vi "get direct child classes.vi"(8 "error in (no error)":errorcluster, 11 "node in":refnum<k20>) -> (0 "error out":errorcluster, 2 "direct child classes":refnum<k20>[](array[refnum]), 3 "node out":refnum<k20>)   [LabVIEW 2023]
uses:
  <vilib>/xml/NI_XML.lvlib
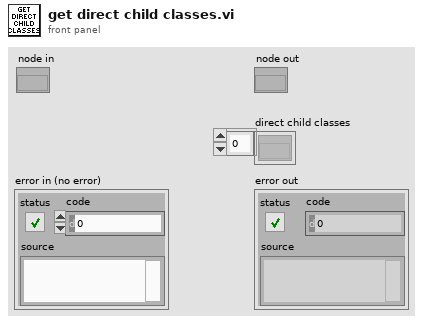
[diagram p1: front panel]
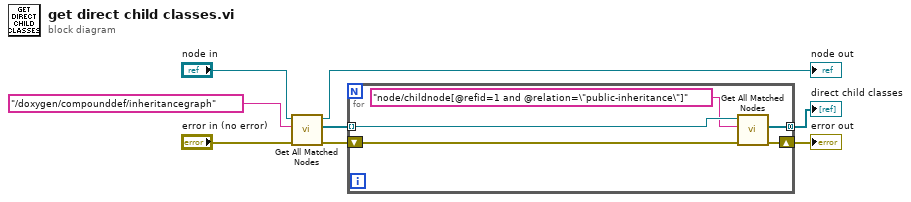
[diagram p0: block diagram]
diagram:
  n1 = call <vilib>:"Get All Matched Nodes.vi"("error in (no error)"="error in (no error)", "XPath expression"="/doxygen/compounddef/inheritancegraph", "node in"="node in") -> ("error out"=w7:errorcluster, "node result array"=w3:refnum<k20>[], "node out"=→"node out":refnum<k20>)  [unwired: 6 in]
  n2 = for {
    tunnel: [w12] -> w6 mode=concatenating
    tunnel: w3 -> [w11] mode=indexing
    shift-right: [w10] -> w8
    shift-left: w7 -> [w13]
    n3 = call <vilib>:"Get All Matched Nodes.vi"("error in (no error)"=w13, "XPath expression"="node/childnode[@refid=1 and @relation=\"public-inheritance\"]", "node in"=w11) -> ("error out"=w10:errorcluster, "node result array"=w12:refnum<k20>[])  [unwired: 6 in, 1 out]
  }
  "error out" <- w8
  "direct child classes" <- w6
